vi "CONEX-LDS Get Low Power Threshold v2.vi"(11 "Connection Cluster in":T1) -> (1 "Left limit":dbl, 3 "Connection Cluster out":T1)   [LabVIEW 2010]
doc: "Get Negative Software Limit"
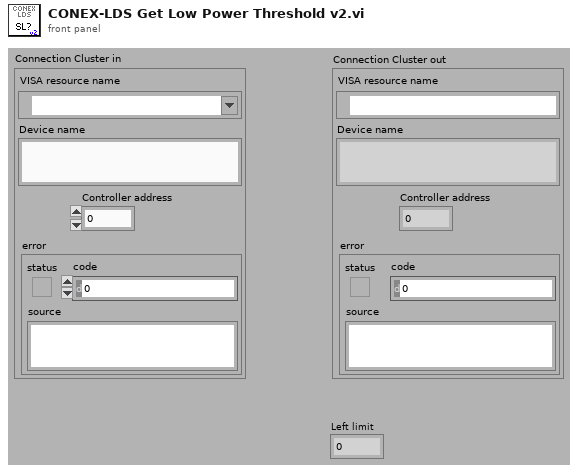
[diagram p1: front panel]
types:
  T1 = cluster{"VISA resource name":refnum<visa-resource-name>, "Device name":string, "Controller address":i32, "error":errorcluster}
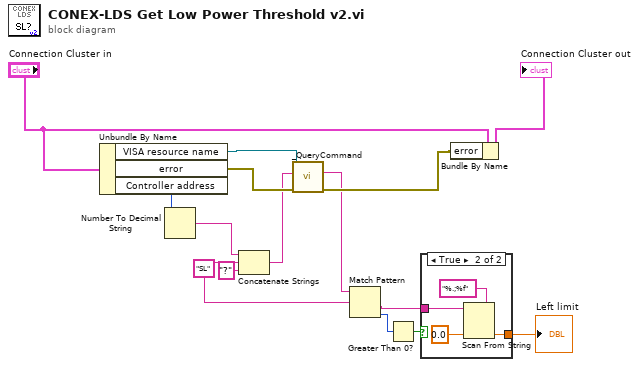
[diagram p0: block diagram]
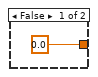
[diagram p2: hidden frame]
diagram:
  w12 = "SL" ("strCommand")
  n1 = Unbundle By Name("Connection Cluster in") -> ("VISA resource name"=w8:refnum<visa-resource-name>, "error"=w6:errorcluster, "Controller address"=w3:i32)
  n2 = Number To Decimal String(number=w3) -> (decimal integer string=w11:string)  [unwired: 1 out]
  n3 = Concatenate Strings(w11, w12, "?" ("strCommand")) -> (w2:string)
  n4 = call <userlib>:"_QueryCommand.vi"("error in"=w6, "Command"=w2, "Instrument Channel in"=w8) -> ("error out"=w7:errorcluster, "Response"=w1:string)  [unwired: 6 in, 1 out]
  n5 = Match Pattern(string=w1, regular expression=w12) -> (after substring=w15:string, offset past match=w14:i32)  [unwired: 3 out]
  n6 = Greater Than 0?(x=w14) -> (x > 0?=w13:bool)
  n7 = case shown="True" w13 {
    tunnel: w15 -> [_ w18]
    tunnel: [0.0 ("valeur par défaut 1") w17] -> w9
    frame False {
    }
    frame True {
      n8 = Scan From String(format string="%.;%f", input string=w18, default 1=0.0 ("valeur par défaut 1")) -> (output 1=w17:dbl)  [unwired: 2 in, 3 out]
    }
  }
  "Left limit" <- w9
  n9 = Bundle By Name(cluster="Connection Cluster in", "error"=w7) -> (→"Connection Cluster out":T1)
